vi "Create TDMS FDMR file.vi"(8 "Sample name":string, 11 "Folder path":path) -> (0 "error out":errorcluster, 3 "tdms map file out":refnum<k34>)   [LabVIEW 2024]
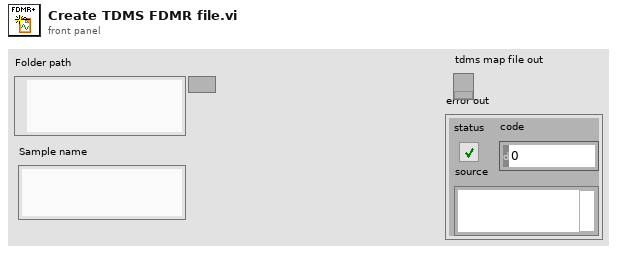
[diagram p1: front panel]
types:
  T1 = enum16{"open", "open or create", "create or replace", "create", "open (read-only)"}
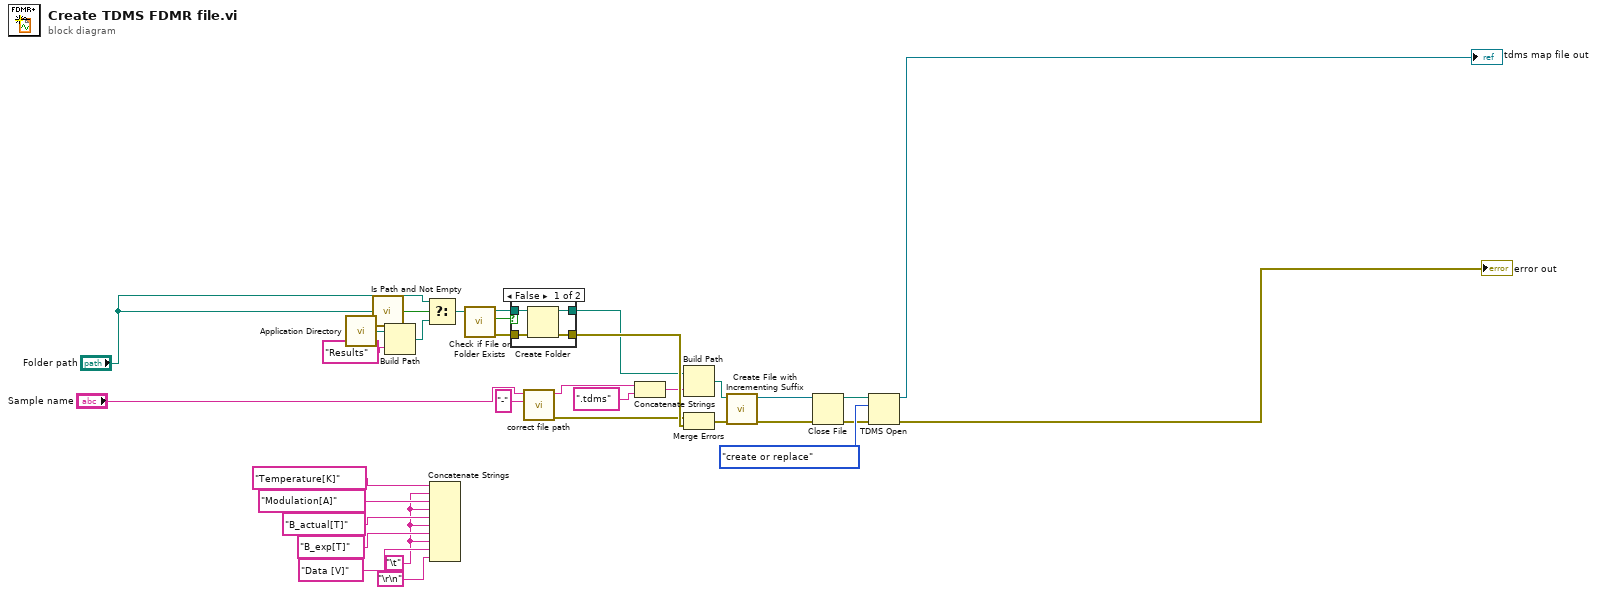
[diagram p0: block diagram]
diagram:
  w25 = "\t"
  n1 = call <vilib>:"Application Directory.vi"() -> ("Application Directory"=w8:path)
  n2 = call <vilib>:"Is Path and Not Empty.vi"("path"="Folder path") -> ("Is Path and Not Empty?"=w17:bool)  [unwired: 4 in]
  n3 = Build Path(base path=w8, name or relative path="Results") -> (appended path=w19:path)
  n4 = Select(t="Folder path", s=w17, f=w19) -> (s? t:f=w18:path)
  n5 = Concatenate Strings("Temperature[K]", w25, "Modulation[A]", w25, "B_actual[T]" ("string"), w25, "B_exp[T]", w25, "Data [V]", "\r\n") -> ()  [unwired: 1 out]
  n6 = call <vilib>:"Check if File or Folder Exists.vi"("path"=w18) -> ("error out"=w15:errorcluster, "file or folder exists?"=w14:bool, "dup path"=w16:path)  [unwired: 8 in]
  n7 = case shown="False" w14 {
    tunnel: w16 -> [w35 w39]
    tunnel: [w36 w38] -> w21
    tunnel: w15 -> [w37 w38]
    tunnel: [w34 w39] -> w20
    frame False {
      n8 = Create Folder(path (use dialog)=w35, error in=w37) -> (created path=w34:path, error out=w36:errorcluster)  [unwired: 1 in, 1 out]
    }
    frame True {
    }
  }
  n9 = call "correct file path.vi"("replacement (-)"="-" ("replacement"), "input path"="Sample name") -> ("error out"=w12:errorcluster, "corrected path"=w9:string)  [unwired: 8 in]
  n10 = Concatenate Strings(w9, ".tdms" ("string")) -> (w10:string)
  n11 = Build Path(base path=w20, name or relative path=w10) -> (appended path=w11:path)
  n12 = Merge Errors(w12, w21) -> (w13:errorcluster)
  n13 = call <vilib>:"Create File with Incrementing Suffix.vi"("error in (no error)"=w13, "file path"=w11) -> ("error out"=w5:errorcluster, "refnum out"=w6:refnum<file>)  [unwired: 7 in, 1 out]
  n14 = Close File(refnum=w6, error in=w5) -> (path=w3:path, error out=w4:errorcluster)
  n15 = TDMS Open(8:w4, 10:T1."create or replace" ("operation (0:open)"), 11:w3) -> (0:→"error out":errorcluster, 3:→"tdms map file out":refnum<k34>)  [unwired: 4 in]
